vi "TouchPanel.Main.vi"(11 "VI ref":refnum<vi>) -> (2 "Label.Text":string, 3 "control used?":bool)   [LabVIEW 2016]
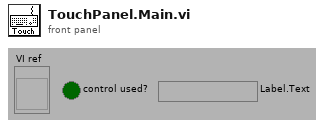
[diagram p1: front panel]
types:
  T1 = typedef "LVNumericRepresentation.ctl" = enum32{"Extended Precision", "Double Precision", "Single Precision", "Long", "Word", "Byte", "Unsigned Long", "Unsigned Word", "Unsigned Byte", "Complex Extended", "Complex Double", "Complex Single", "Quad", "Unsigned Quad", "Fixed-Point"}
  T2 = typedef "LVRowAndColumnTypeDef.ctl" = cluster{"Row":i32, "Column":i32}
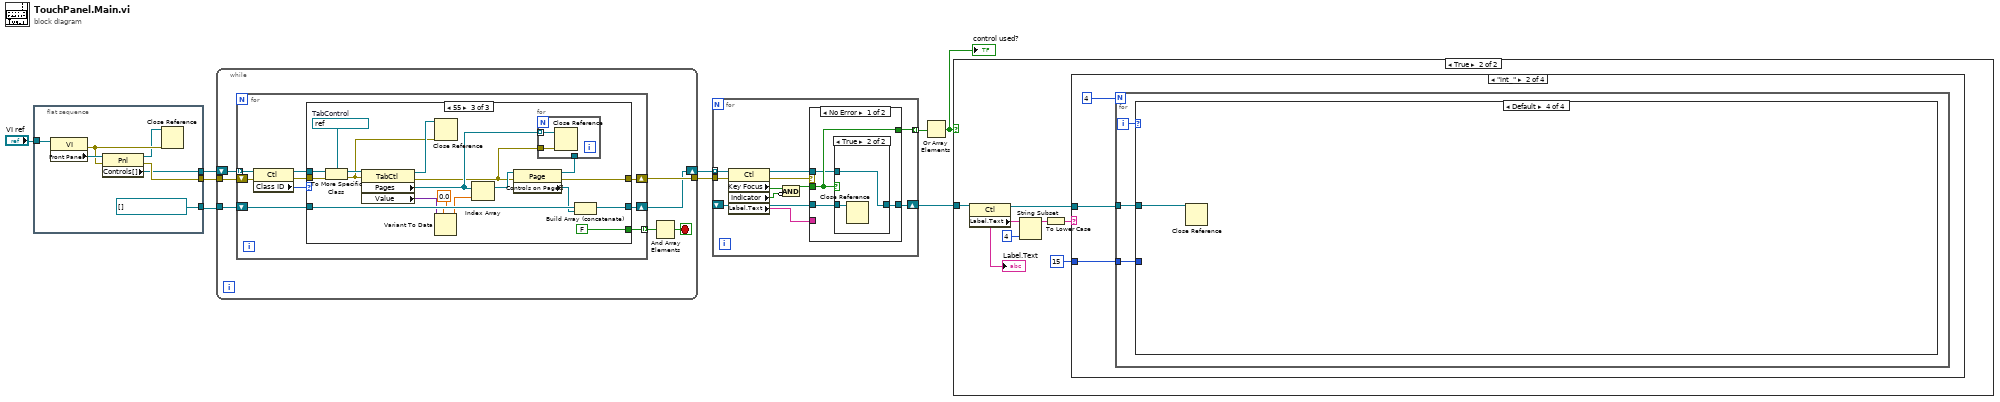
[diagram p0: block diagram]
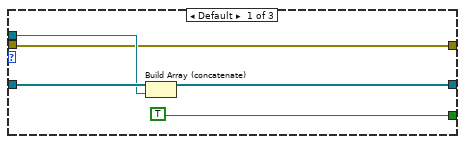
[diagram p2: hidden frame]
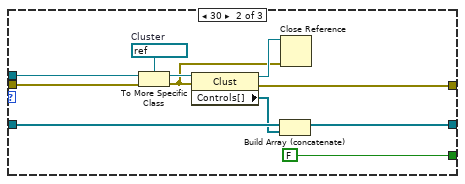
[diagram p3: hidden frame]
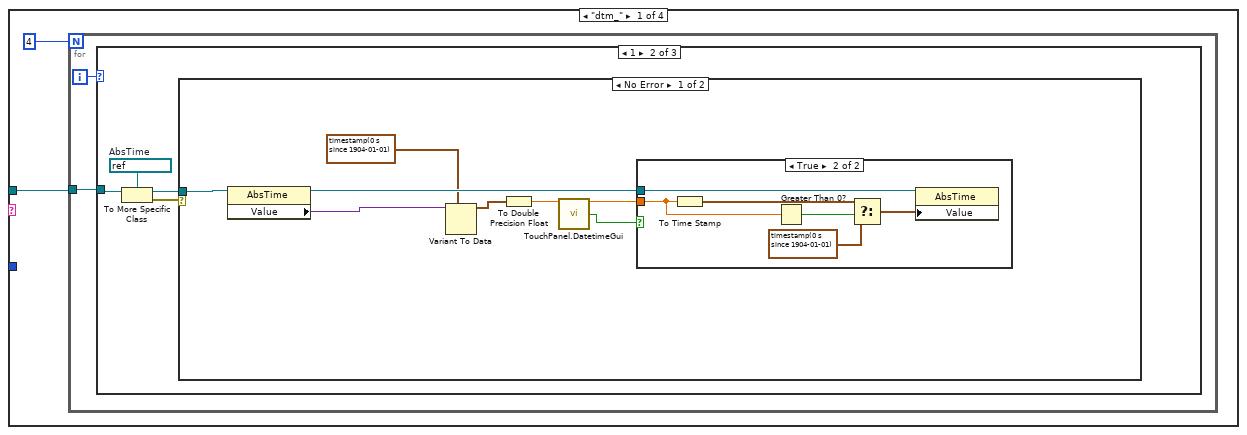
[diagram p5: hidden frame]
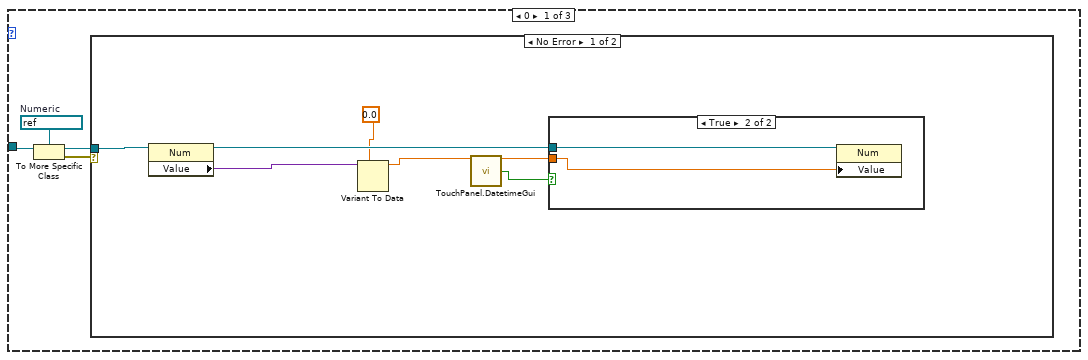
[diagram p6: hidden frame]
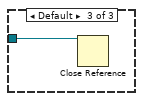
[diagram p11: hidden frame]
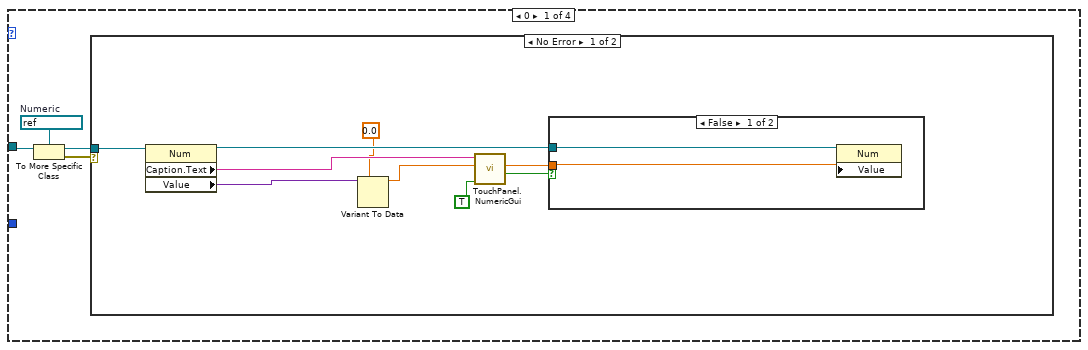
[diagram p12: hidden frame]
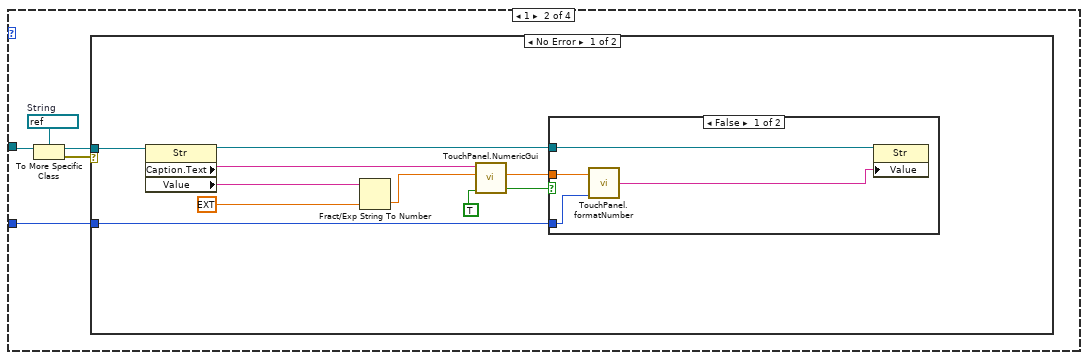
[diagram p15: hidden frame]
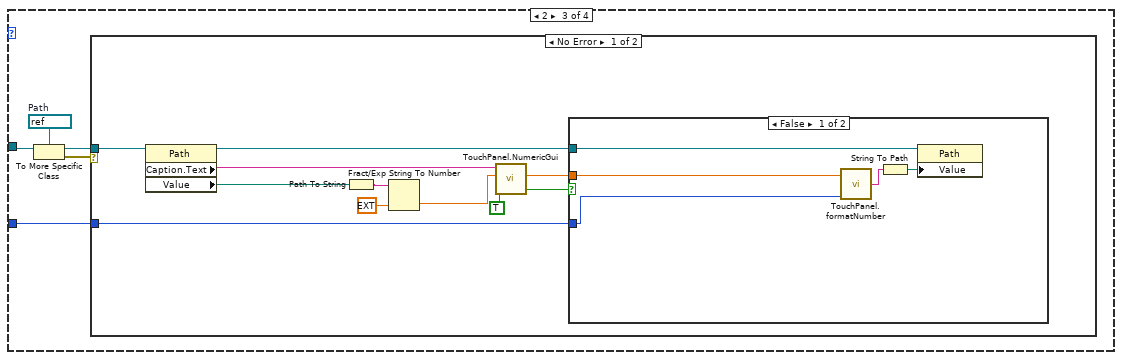
[diagram p18: hidden frame]
diagram:
  n1 = flat-sequence {
    tunnel: [w13] -> w7
    tunnel: [refnum<vi>[] []] -> w5
    tunnel: [w11] -> w4
    tunnel: "VI ref" -> [w10]
    frame #0 {
      n2 = property class="VI"(reference=w10) -> (error out=w15:errorcluster, "Front Panel"=w16:refnum<vi>)  [unwired: 1 in, 1 out]
      n3 = property class="Pnl"(reference=w16, error in=w15) -> (reference out=w14:refnum<vi>, error out=w13:errorcluster, "Controls[]"=w11:refnum<vi>[])
      n4 = Close Reference(reference=w14, error in (no error)=w15) -> ()  [unwired: 1 out]
    }
  }
  n5 = while {
    tunnel: w7 -> [w23]
    tunnel: [w22] -> w6
    tunnel: w5 -> [w21]
    shift-right: [w19] -> w3
    shift-left: w4 -> [w20]
    stop <- w17 stop-if-true
    n6 = for {
      tunnel: w20 -> [w32] mode=indexing
      shift-right: [w26] -> w22
      shift-left: w23 -> [w31]
      shift-right: [w27] -> w19
      shift-left: w21 -> [w28]
      tunnel: [w24] -> w18 mode=indexing
      n7 = property class="Ctl"(reference=w32, error in=w31) -> (reference out=w30:refnum<vi>, error out=w29:errorcluster, "Class ID"=w25:u32)
      n8 = case shown="55" w25 {
        tunnel: w30 -> [w36 w46 w65]
        tunnel: w29 -> [w34 w45 w64]
        tunnel: w28 -> [w37 w42 w60]
        tunnel: [w35 w40 w59] -> w27
        tunnel: [w34 w39 w58] -> w26
        tunnel: [TRUE FALSE FALSE] -> w24
        frame Default {
          n9 = Build Array (concatenate)(w37, w36) -> (w35:refnum<vi>[])
        }
        frame 30 {
          w47 = refnum<vi> refnum  # Cluster
          n10 = To More Specific Class(target class=w47, reference=w46, error in=w45) -> (specific class reference=w48:refnum<vi>, error out=w43:errorcluster)
          n11 = property class="Clust"(reference=w48, error in=w43) -> (reference out=w44:refnum<vi>, error out=w39:errorcluster, "Controls[]"=w41:refnum<vi>[])
          n12 = Build Array (concatenate)(w42, w41) -> (w40:refnum<vi>[])
          n13 = Close Reference(reference=w44, error in (no error)=w43) -> ()  [unwired: 1 out]
        }
        frame 55 {
          w61 = refnum<vi> refnum  # TabControl
          n14 = To More Specific Class(target class=w61, reference=w65, error in=w64) -> (specific class reference=w66:refnum<vi>, error out=w62:errorcluster)
          n15 = property class="TabCtl"(reference=w66, error in=w62) -> (reference out=w63:refnum<vi>, error out=w50:errorcluster, "Pages"=w51:refnum<vi>[], "Value"=w56:variant)
          n16 = Variant To Data(type=0.0 ("value"), Variant=w56) -> (data=w54:dbl)  [unwired: 1 in, 1 out]
          n17 = Close Reference(reference=w63, error in (no error)=w62) -> ()  [unwired: 1 out]
          n18 = Index Array(array=w51, index=w54) -> (element=w53:refnum<vi>)
          n19 = property class="Page"(reference=w53, error in=w50) -> (reference out=w49:refnum<vi>, error out=w58:errorcluster, "Controls on Page[]"=w52:refnum<vi>[])
          n20 = for {
            tunnel: w51 -> [w68] mode=indexing
            tunnel: w50 -> [w67]
            tunnel: w49 -> [_]
            n21 = Close Reference(reference=w68, error in (no error)=w67) -> ()  [unwired: 1 out]
          }
          n22 = Build Array (concatenate)(w60, w52) -> (w59:refnum<vi>[])
        }
      }
    }
    n23 = And Array Elements(Boolean array=w18) -> (logical AND=w17:bool)
  }
  n24 = for {
    tunnel: w3 -> [w79] mode=indexing
    shift-right: [w74] -> w8
    shift-left: _ -> [w76]
    tunnel: w6 -> [w78]
    tunnel: [w73] -> w9 mode=indexing
    n25 = property class="Ctl"(reference=w79, error in=w78) -> (reference out=w77:refnum<vi>, error out=w75:errorcluster, "Key Focus"=w71:bool, "Indicator"=w70:bool, "Label.Text"=w69:string)
    n26 = Compound Arithmetic op=AND(w71, invert w70) -> (w72:bool)
    n27 = case shown="No Error" w75 {
      tunnel: w77 -> [w82 _]
      tunnel: w76 -> [w81 w89]
      tunnel: w72 -> [w83 _]
      tunnel: [w80 w89] -> w74
      tunnel: [w83 FALSE ("Key Focus")] -> w73
      tunnel: w69 -> [_ _]
      frame No Error {
        n28 = case shown="True" w83 {
          tunnel: w82 -> [w85 w86]
          tunnel: w81 -> [w84 w87]
          tunnel: [w84 w86] -> w80
          frame False {
            n29 = Close Reference(reference=w85) -> ()  [unwired: 1 in, 1 out]
          }
          frame True {
            n30 = Close Reference(reference=w87) -> ()  [unwired: 1 in, 1 out]
          }
        }
      }
      frame Error {
      }
    }
  }
  n31 = Or Array Elements(Boolean array=w9) -> (logical OR=w2:bool)
  "control used?" <- w2
  n32 = case shown="True" w2 {
    tunnel: w8 -> [_ w96]
    frame False {
    }
    frame True {
      n33 = property class="Ctl"(reference=w96) -> (reference out=w95:refnum<vi>, "Label.Text"=w90:string)  [unwired: 1 in, 1 out]
      "Label.Text" <- w90
      n34 = String Subset(string=w90, length (rest)=4 ("length (rest)")) -> (substring=w94:string)  [unwired: 1 out]
      n35 = To Lower Case(string=w94) -> (all lower case string=w92:string)
      n36 = case shown="\"int_\"" w92 {
        selector: w92 -> [_ _ _ w259]
        tunnel: w95 -> [w97 w134 w196 w261]
        tunnel: i16 15 ("significant digits (6)") -> [_ w133 w195 _]
        frame "dtm_" {
          n37 = for {
            N: 4 -> [_]
            tunnel: w97 -> [w100]
            i -> [w99]
            n38 = case shown="1" w99 {
              tunnel: w100 -> [w101 w114 w132]
              frame 0 {
                w104 = refnum<vi> refnum  # Numeric
                n39 = To More Specific Class(target class=w104, reference=w101) -> (specific class reference=w102:refnum<vi>, error out=w103:errorcluster)  [unwired: 1 in]
                n40 = case shown="No Error" w103 {
                  tunnel: w102 -> [w111 _]
                  frame No Error {
                    n41 = property class="Num"(reference=w111) -> (reference out=w110:refnum<vi>, "Value"=w109:variant)  [unwired: 1 in, 1 out]
                    n42 = Variant To Data(type=0.0 ("value"), Variant=w109) -> (data=w107:dbl)  [unwired: 1 in, 1 out]
                    n43 = call "TouchPanel.DatetimeGui.vi"("num date/time in (now)"=w107) -> ("num date/time out"=w106:dbl, "ok"=w105:bool)  [unwired: 1 in, 12 out]
                    n44 = case shown="True" w105 {
                      tunnel: w110 -> [_ w113]
                      tunnel: w106 -> [_ w112]
                      frame False {
                      }
                      frame True {
                        n45 = property class="Num"(reference=w113, "Value"=w112) -> ()  [unwired: 1 in, 2 out]
                      }
                    }
                  }
                  frame Error {
                  }
                }
              }
              frame 1 {
                w117 = refnum<vi> refnum  # AbsTime
                n46 = To More Specific Class(target class=w117, reference=w114) -> (specific class reference=w115:refnum<vi>, error out=w116:errorcluster)  [unwired: 1 in]
                n47 = case shown="No Error" w116 {
                  tunnel: w115 -> [w125 _]
                  frame No Error {
                    n48 = property class="AbsTime"(reference=w125) -> (reference out=w124:refnum<vi>, "Value"=w123:variant)  [unwired: 1 in, 1 out]
                    n49 = Variant To Data(type=timestamp(0 s since 1904-01-01), Variant=w123) -> (data=w122:timestamp)  [unwired: 1 in, 1 out]
                    n50 = To Double Precision Float(number=w122) -> (double precision float=w118:dbl)
                    n51 = call "TouchPanel.DatetimeGui.vi"("num date/time in (now)"=w118) -> ("num date/time out"=w121:dbl, "ok"=w120:bool)  [unwired: 1 in, 12 out]
                    n52 = case shown="True" w120 {
                      tunnel: w124 -> [_ w131]
                      tunnel: w121 -> [_ w127]
                      frame False {
                      }
                      frame True {
                        n53 = To Time Stamp(1:w127) -> (0:w129:timestamp)
                        n54 = Greater Than 0?(x=w127) -> (x > 0?=w130:bool)
                        n55 = Select(t=w129, s=w130, f=timestamp(0 s since 1904-01-01) ("time stamp")) -> (s? t:f=w128:timestamp)
                        n56 = property class="AbsTime"(reference=w131, "Value"=w128) -> ()  [unwired: 1 in, 2 out]
                      }
                    }
                  }
                  frame Error {
                  }
                }
              }
              frame Default {
                n57 = Close Reference(reference=w132) -> ()  [unwired: 1 in, 1 out]
              }
            }
          }
        }
        frame "int_" {
          n58 = for {
            N: 4 -> [_]
            tunnel: w134 -> [w138]
            tunnel: w133 -> [w136]
            i -> [w137]
            n59 = case shown="Default" w137 {
              tunnel: w138 -> [w139 w156 w175 w194]
              tunnel: w136 -> [_ w154 w173 _]
              frame 0 {
                w142 = refnum<vi> refnum  # Numeric
                n60 = To More Specific Class(target class=w142, reference=w139) -> (specific class reference=w140:refnum<vi>, error out=w141:errorcluster)  [unwired: 1 in]
                n61 = case shown="No Error" w141 {
                  tunnel: w140 -> [w151 _]
                  frame No Error {
                    n62 = property class="Num"(reference=w151) -> (reference out=w150:refnum<vi>, "Caption.Text"=w148:string, "Value"=w149:variant)  [unwired: 1 in, 1 out]
                    n63 = Variant To Data(type=0.0 ("value"), Variant=w149) -> (data=w145:dbl)  [unwired: 1 in, 1 out]
                    n64 = call "TouchPanel.NumericGui.vi"("Integer (F)"=TRUE, "Numeric In"=w145, "Message In"=w148) -> ("Canceled"=w146:bool, "Numeric Out"=w144:ext)  [unwired: 3 in, 4 out]
                    n65 = case shown="False" w146 {
                      tunnel: w150 -> [w153 _]
                      tunnel: w144 -> [w152 _]
                      frame False {
                        n66 = property class="Num"(reference=w153, "Value"=w152) -> ()  [unwired: 1 in, 2 out]
                      }
                      frame True {
                      }
                    }
                  }
                  frame Error {
                  }
                }
              }
              frame 1 {
                w155 = refnum<vi> refnum  # String
                n67 = To More Specific Class(target class=w155, reference=w156) -> (specific class reference=w157:refnum<vi>, error out=w158:errorcluster)  [unwired: 1 in]
                n68 = case shown="No Error" w158 {
                  tunnel: w157 -> [w168 _]
                  tunnel: w154 -> [w159 _]
                  frame No Error {
                    n69 = property class="Str"(reference=w168) -> (reference out=w167:refnum<vi>, "Caption.Text"=w164:string, "Value"=w166:string)  [unwired: 1 in, 1 out]
                    n70 = Fract/Exp String To Number(string=w166, default (0 dbl)=ext 0.0 ("default (0 DBL)")) -> (number=w163:ext)  [unwired: 1 in, 2 out]
                    n71 = call "TouchPanel.NumericGui.vi"("Integer (F)"=TRUE, "Numeric In"=w163, "Message In"=w164) -> ("Canceled"=w162:bool, "Numeric Out"=w161:ext)  [unwired: 3 in, 4 out]
                    n72 = case shown="False" w162 {
                      tunnel: w167 -> [w172 _]
                      tunnel: w161 -> [w171 _]
                      tunnel: w159 -> [w169 _]
                      frame False {
                        n73 = call "TouchPanel.formatNumber.vi"("number in"=w171, "significant digits (6)"=w169) -> ("string out"=w170:string)  [unwired: 2 in, 11 out]
                        n74 = property class="Str"(reference=w172, "Value"=w170) -> ()  [unwired: 1 in, 2 out]
                      }
                      frame True {
                      }
                    }
                  }
                  frame Error {
                  }
                }
              }
              frame 2 {
                w174 = refnum<vi> refnum  # Path
                n75 = To More Specific Class(target class=w174, reference=w175) -> (specific class reference=w176:refnum<vi>, error out=w177:errorcluster)  [unwired: 1 in]
                n76 = case shown="No Error" w177 {
                  tunnel: w176 -> [w188 _]
                  tunnel: w173 -> [w178 _]
                  frame No Error {
                    n77 = property class="Path"(reference=w188) -> (reference out=w182:refnum<vi>, "Caption.Text"=w181:string, "Value"=w180:path)  [unwired: 1 in, 1 out]
                    n78 = Path To String(path=w180) -> (string=w187:string)
                    n79 = Fract/Exp String To Number(string=w187, default (0 dbl)=ext 0.0 ("default (0 DBL)")) -> (number=w185:ext)  [unwired: 1 in, 2 out]
                    n80 = call "TouchPanel.NumericGui.vi"("Integer (F)"=TRUE, "Numeric In"=w185, "Message In"=w181) -> ("Canceled"=w184:bool, "Numeric Out"=w183:ext)  [unwired: 3 in, 4 out]
                    n81 = case shown="False" w184 {
                      tunnel: w182 -> [w193 _]
                      tunnel: w183 -> [w192 _]
                      tunnel: w178 -> [w189 _]
                      frame False {
                        n82 = call "TouchPanel.formatNumber.vi"("number in"=w192, "significant digits (6)"=w189) -> ("string out"=w191:string)  [unwired: 2 in, 11 out]
                        n83 = String To Path(string=w191) -> (path=w190:path)
                        n84 = property class="Path"(reference=w193, "Value"=w190) -> ()  [unwired: 1 in, 2 out]
                      }
                      frame True {
                      }
                    }
                  }
                  frame Error {
                  }
                }
              }
              frame Default {
                n85 = Close Reference(reference=w194) -> ()  [unwired: 1 in, 1 out]
              }
            }
          }
        }
        frame "num_" {
          n86 = for {
            N: 4 -> [_]
            tunnel: w196 -> [w200]
            tunnel: w195 -> [w198]
            i -> [w199]
            n87 = case shown="2" w199 {
              tunnel: w200 -> [w201 w221 w239 w257]
              tunnel: w198 -> [_ w219 w237 _]
              frame 0 {
                w204 = refnum<vi> refnum  # Numeric
                n88 = To More Specific Class(target class=w204, reference=w201) -> (specific class reference=w202:refnum<vi>, error out=w203:errorcluster)  [unwired: 1 in]
                n89 = case shown="No Error" w203 {
                  tunnel: w202 -> [w216 _]
                  frame No Error {
                    n90 = property class="Num"(reference=w216) -> (reference out=w215:refnum<vi>, "Caption.Text"=w213:string, "Value"=w214:variant, "Representation"=w208:T1)  [unwired: 1 in, 1 out]
                    n91 = Variant To Data(type=0.0 ("value"), Variant=w214) -> (data=w210:dbl)  [unwired: 1 in, 1 out]
                    n92 = In Range and Coerce(upper limit=u32 8, x=w208, lower limit=u32 3 ("upper limit")) -> (In Range?=w207:bool)  [unwired: 1 out]
                    n93 = call "TouchPanel.NumericGui.vi"("Integer (F)"=w207, "Numeric In"=w210, "Message In"=w213) -> ("Canceled"=w211:bool, "Numeric Out"=w209:ext)  [unwired: 3 in, 4 out]
                    n94 = case shown="False" w211 {
                      tunnel: w215 -> [w218 _]
                      tunnel: w209 -> [w217 _]
                      frame False {
                        n95 = property class="Num"(reference=w218, "Value"=w217) -> ()  [unwired: 1 in, 2 out]
                      }
                      frame True {
                      }
                    }
                  }
                  frame Error {
                  }
                }
              }
              frame 1 {
                w220 = refnum<vi> refnum  # String
                n96 = To More Specific Class(target class=w220, reference=w221) -> (specific class reference=w222:refnum<vi>, error out=w223:errorcluster)  [unwired: 1 in]
                n97 = case shown="No Error" w223 {
                  tunnel: w222 -> [w232 _]
                  tunnel: w219 -> [w224 _]
                  frame No Error {
                    n98 = property class="Str"(reference=w232) -> (reference out=w231:refnum<vi>, "Caption.Text"=w228:string, "Value"=w230:string)  [unwired: 1 in, 1 out]
                    n99 = Fract/Exp String To Number(string=w230, default (0 dbl)=ext 0.0 ("default (0 DBL)")) -> (number=w227:ext)  [unwired: 1 in, 2 out]
                    n100 = call "TouchPanel.NumericGui.vi"("Numeric In"=w227, "Message In"=w228) -> ("Canceled"=w226:bool, "Numeric Out"=w225:ext)  [unwired: 4 in, 4 out]
                    n101 = case shown="False" w226 {
                      tunnel: w231 -> [w236 _]
                      tunnel: w225 -> [w235 _]
                      tunnel: w224 -> [w233 _]
                      frame False {
                        n102 = call "TouchPanel.formatNumber.vi"("number in"=w235, "significant digits (6)"=w233) -> ("string out"=w234:string)  [unwired: 2 in, 11 out]
                        n103 = property class="Str"(reference=w236, "Value"=w234) -> ()  [unwired: 1 in, 2 out]
                      }
                      frame True {
                      }
                    }
                  }
                  frame Error {
                  }
                }
              }
              frame 2 {
                w238 = refnum<vi> refnum  # Path
                n104 = To More Specific Class(target class=w238, reference=w239) -> (specific class reference=w240:refnum<vi>, error out=w241:errorcluster)  [unwired: 1 in]
                n105 = case shown="No Error" w241 {
                  tunnel: w240 -> [w251 _]
                  tunnel: w237 -> [w242 _]
                  frame No Error {
                    n106 = property class="Path"(reference=w251) -> (reference out=w245:refnum<vi>, "Caption.Text"=w244:string, "Value"=w243:path)  [unwired: 1 in, 1 out]
                    n107 = Path To String(path=w243) -> (string=w250:string)
                    n108 = Fract/Exp String To Number(string=w250, default (0 dbl)=ext 0.0 ("default (0 DBL)")) -> (number=w248:ext)  [unwired: 1 in, 2 out]
                    n109 = call "TouchPanel.NumericGui.vi"("Numeric In"=w248, "Message In"=w244) -> ("Canceled"=w247:bool, "Numeric Out"=w246:ext)  [unwired: 4 in, 4 out]
                    n110 = case shown="False" w247 {
                      tunnel: w245 -> [w256 _]
                      tunnel: w246 -> [w255 _]
                      tunnel: w242 -> [w252 _]
                      frame False {
                        n111 = call "TouchPanel.formatNumber.vi"("number in"=w255, "significant digits (6)"=w252) -> ("string out"=w254:string)  [unwired: 2 in, 11 out]
                        n112 = String To Path(string=w254) -> (path=w253:path)
                        n113 = property class="Path"(reference=w256, "Value"=w253) -> ()  [unwired: 1 in, 2 out]
                      }
                      frame True {
                      }
                    }
                  }
                  frame Error {
                  }
                }
              }
              frame Default {
                n114 = Close Reference(reference=w257) -> ()  [unwired: 1 in, 1 out]
              }
            }
          }
        }
        frame Default {
          n115 = Equal?(x=w259, y="pwd_") -> (x = y?=w260:bool)
          n116 = for {
            N: 5 -> [_]
            tunnel: w261 -> [w265]
            tunnel: w260 -> [w263]
            i -> [w264]
            n117 = case shown="1" w264 {
              tunnel: w265 -> [w267 w287 w302 w318 w365]
              tunnel: w263 -> [w266 w285 w300 w317 _]
              frame 0 {
                w270 = refnum<vi> refnum  # Numeric
                n118 = To More Specific Class(target class=w270, reference=w267) -> (specific class reference=w268:refnum<vi>, error out=w269:errorcluster)  [unwired: 1 in]
                n119 = case shown="No Error" w269 {
                  tunnel: w268 -> [w271 _]
                  tunnel: w266 -> [w276 _]
                  frame No Error {
                    n120 = property class="Num"(reference=w271) -> ("Caption.Text"=w281:string, "Value"=w282:variant, "Representation"=w273:T1)  [unwired: 1 in, 2 out]
                    n121 = Variant To Data(type=0.0 ("value"), Variant=w282) -> (data=w278:dbl)  [unwired: 1 in, 1 out]
                    n122 = In Range and Coerce(upper limit=u32 8, x=w273, lower limit=u32 3 ("upper limit")) -> (In Range?=w272:bool)  [unwired: 1 out]
                    n123 = call "TouchPanel.NumericGui.vi"("Password Display (F)"=w276, "Integer (F)"=w272, "Numeric In"=w278, "Message In"=w281) -> ("Canceled"=w279:bool, "Numeric Out"=w277:ext)  [unwired: 2 in, 4 out]
                    n124 = case shown="False" w279 {
                      tunnel: w271 -> [w284 _]
                      tunnel: w277 -> [w283 _]
                      frame False {
                        n125 = property class="Num"(reference=w284, "Val(Sgnl)"=w283) -> ()  [unwired: 1 in, 2 out]
                      }
                      frame True {
                      }
                    }
                  }
                  frame Error {
                  }
                }
              }
              frame 1 {
                w286 = refnum<vi> refnum  # String
                n126 = To More Specific Class(target class=w286, reference=w287) -> (specific class reference=w288:refnum<vi>, error out=w289:errorcluster)  [unwired: 1 in]
                n127 = case shown="No Error" w289 {
                  tunnel: w288 -> [w297 _]
                  tunnel: w285 -> [w291 _]
                  frame No Error {
                    n128 = property class="Str"(reference=w297) -> (reference out=w296:refnum<vi>, "Caption.Text"=w294:string, "Value"=w295:string, "Limit To Single Line?"=w290:bool)  [unwired: 1 in, 1 out]
                    n129 = call "TouchPanel.AlphanumericGui.vi"("Password Display (F)"=w291, "Limit to single line (T)"=w290, "String In"=w295, "Message In"=w294) -> ("Canceled"=w292:bool, "String Out"=w293:string)  [unwired: 1 in, 5 out]
                    n130 = case shown="False" w292 {
                      tunnel: w296 -> [w299 _]
                      tunnel: w293 -> [w298 _]
                      frame False {
                        n131 = property class="Str"(reference=w299, "Val(Sgnl)"=w298) -> ()  [unwired: 1 in, 2 out]
                      }
                      frame True {
                      }
                    }
                  }
                  frame Error {
                  }
                }
              }
              frame 2 {
                w301 = refnum<vi> refnum  # Path
                n132 = To More Specific Class(target class=w301, reference=w302) -> (specific class reference=w303:refnum<vi>, error out=w304:errorcluster)  [unwired: 1 in]
                n133 = case shown="No Error" w304 {
                  tunnel: w303 -> [w313 _]
                  tunnel: w300 -> [w305 _]
                  frame No Error {
                    n134 = property class="Path"(reference=w313) -> (reference out=w312:refnum<vi>, "Caption.Text"=w309:string, "Value"=w311:path)  [unwired: 1 in, 1 out]
                    n135 = Path To String(path=w311) -> (string=w308:string)
                    n136 = call "TouchPanel.AlphanumericGui.vi"("Password Display (F)"=w305, "String In"=w308, "Message In"=w309) -> ("Canceled"=w307:bool, "String Out"=w306:string)  [unwired: 2 in, 5 out]
                    n137 = String To Path(string=w306) -> (path=w310:path)
                    n138 = case shown="False" w307 {
                      tunnel: w312 -> [w315 _]
                      tunnel: w310 -> [w314 _]
                      frame False {
                        n139 = property class="Path"(reference=w315, "Val(Sgnl)"=w314) -> ()  [unwired: 1 in, 2 out]
                      }
                      frame True {
                      }
                    }
                  }
                  frame Error {
                  }
                }
              }
              frame 3 {
                n140 = To More Specific Class(target class=refnum<vi> refnum ("Table"), reference=w318) -> (specific class reference=w319:refnum<vi>, error out=w320:errorcluster)  [unwired: 1 in]
                n141 = case shown="No Error" w320 {
                  tunnel: w319 -> [w332 _]
                  tunnel: w317 -> [w330 _]
                  frame No Error {
                    n142 = property class="Tbl (strict)" props=["Row Headers[]", "Column Headers[]", "Caption", "Text", "Value", "EditPos"](reference=w332) -> (reference out=w331:refnum<vi>, "Row Headers[]"=w328:string[], "Column Headers[]"=w327:string[], "Value"=w325:string[][], "EditPos"=w329:T2)  [unwired: 1 in, 2 out]
                    n143 = Array Size(array=w325) -> (size(s)=w324:i32[])
                    n144 = Unbundle(w329) -> ("Row"=w322:i32, "Column"=w326:i32)
                    n145 = Index Array(array=w324) -> (element=w323:i32)  [unwired: 1 in]
                    n146 = Less?(x=w322, y=w323) -> (x < y?=w321:bool)
                    n147 = case shown="True" w321 {
                      tunnel: w331 -> [_ w355]
                      tunnel: w330 -> [_ w354]
                      tunnel: w329 -> [_ w349]
                      tunnel: w328 -> [_ w347]
                      tunnel: w327 -> [_ w346]
                      tunnel: w326 -> [_ w345]
                      tunnel: w325 -> [_ w340]
                      tunnel: w322 -> [_ w339]
                      frame False {
                      }
                      frame True {
                        n148 = Index Array(array=w346, index=w345) -> (element=w343:string)
                        n149 = Index Array(array=w347, index=w339) -> (element=w344:string)
                        n150 = Index Array(array=w340, index (row)=w339, index (col)=w345) -> (element=w352:string)
                        n151 = Concatenate Strings(w344, " - ", w343) -> (w341:string)
                        n152 = Fract/Exp String To Number(string=w352, default (0 dbl)=ext 0.0 ("default (0 DBL)")) -> (number=w350:ext)  [unwired: 1 in, 2 out]
                        n153 = call "TouchPanel.NumericGui.vi"("Password Display (F)"=w354, "empty visible (F)"=TRUE, "Numeric In"=w350, "Message In"=w341) -> ("Canceled"=w353:bool, "Numeric Out"=w338:ext)  [unwired: 2 in, 4 out]
                        n154 = Number To Fractional String(number=w338, precision (6)=i16 9) -> (F-format string=w336:string)  [unwired: 1 in, 1 out]
                        n155 = Not A Number/Path/Refnum?(number/path/refnum=w338) -> (NaN/Path/Refnum?=w337:bool)
                        n156 = Select(t="", s=w337, f=w336) -> (s? t:f=w334:string)
                        n157 = case shown="False" w353 {
                          tunnel: w355 -> [w364 _]
                          tunnel: w334 -> [w357 _]
                          tunnel: w349 -> [w356 _]
                          frame False {
                            n158 = property class="Tbl (strict)"(reference=w364) -> (reference out=w363:refnum<vi>, error out=w362:errorcluster, "Value"=w361:string[][])  [unwired: 1 in]
                            n159 = Unbundle(w356) -> ("Row"=w359:i32, "Column"=w358:i32)
                            n160 = Replace Array Subset(array=w361, new element=w357, index (row)=w359, index (col)=w358) -> (w360:string[][])
                            n161 = property class="Tbl (strict)"(reference=w363, error in=w362, "Val(Sgnl)"=w360) -> ()  [unwired: 2 out]
                          }
                          frame True {
                          }
                        }
                      }
                    }
                  }
                  frame Error {
                  }
                }
              }
              frame Default {
                n162 = Close Reference(reference=w365) -> ()  [unwired: 1 in, 1 out]
              }
            }
          }
        }
      }
    }
  }
